vi "Untitled 1.vi"() -> ()   [LabVIEW 2023]
panel:
  in  "Restart":bool
  in  "8 8":string
  in  "7 8":string
  in  "6 8":string="2"
  in  "5 8":string="7"
  in  "8 7":string
  in  "7 7":string
  in  "6 7":string
  in  "5 7":string="8"
  in  "8 6":string
  in  "7 6":string
  in  "6 6":string
  in  "5 6":string="1"
  in  "8 5":string="5"
  in  "7 5":string
  in  "6 5":string
  in  "5 5":string
  in  "8 4":string="4"
  in  "7 4":string="3"
  in  "6 4":string="7"
  in  "5 4":string
  in  "8 3":string
  in  "7 3":string="8"
  in  "6 3":string
  in  "5 3":string="2"
  in  "8 2":string
  in  "7 2":string
  in  "6 2":string="4"
  in  "5 2":string="6"
  in  "8 1":string="1"
  in  "7 1":string="7"
  in  "6 1":string
  in  "5 1":string
  in  "8 0":string="8"
  in  "7 0":string="6"
  in  "6 0":string="9"
  in  "5 0":string
  in  "4 8":string
  in  "4 7":string="9"
  in  "4 6":string
  in  "4 5":string
  in  "4 4":string
  in  "4 3":string
  in  "4 2":string="3"
  in  "4 1":string
  in  "4 0":string
  in  "3 8":string="4"
  in  "3 7":string
  in  "3 6":string
  in  "3 5":string
  in  "3 4":string
  in  "3 3":string="6"
  in  "3 2":string="8"
  in  "3 1":string="5"
  in  "3 0":string
  in  "2 8":string
  in  "2 7":string="1"
  in  "2 6":string
  in  "2 5":string="7"
  in  "2 4":string
  in  "2 3":string
  in  "2 2":string
  in  "2 1":string
  in  "2 0":string
  in  "1 8":string="9"
  in  "1 7":string
  in  "1 6":string="3"
  in  "1 5":string
  in  "1 4":string="6"
  in  "1 3":string
  in  "1 2":string
  in  "1 1":string
  in  "1 0":string="2"
  in  "0 8":string="5"
  in  "0 7":string
  in  "0 6":string="6"
  in  "0 5":string="1"
  in  "0 4":string="9"
  in  "0 3":string="4"
  in  "0 2":string="7"
  in  "0 1":string
  in  "0 0":string
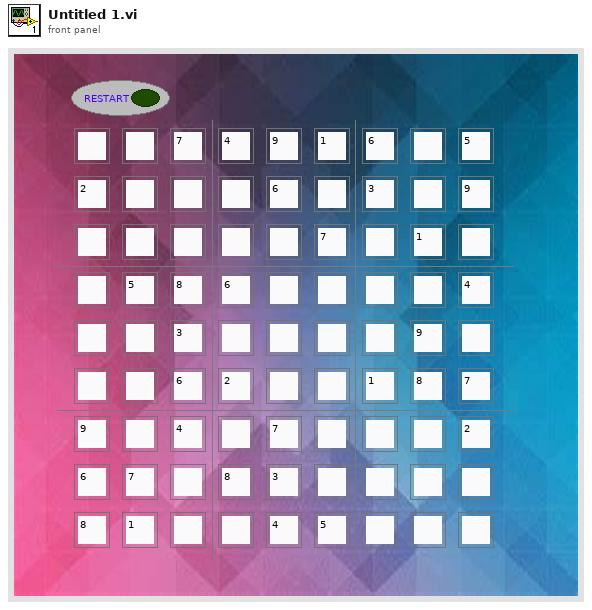
[diagram p1: front panel]
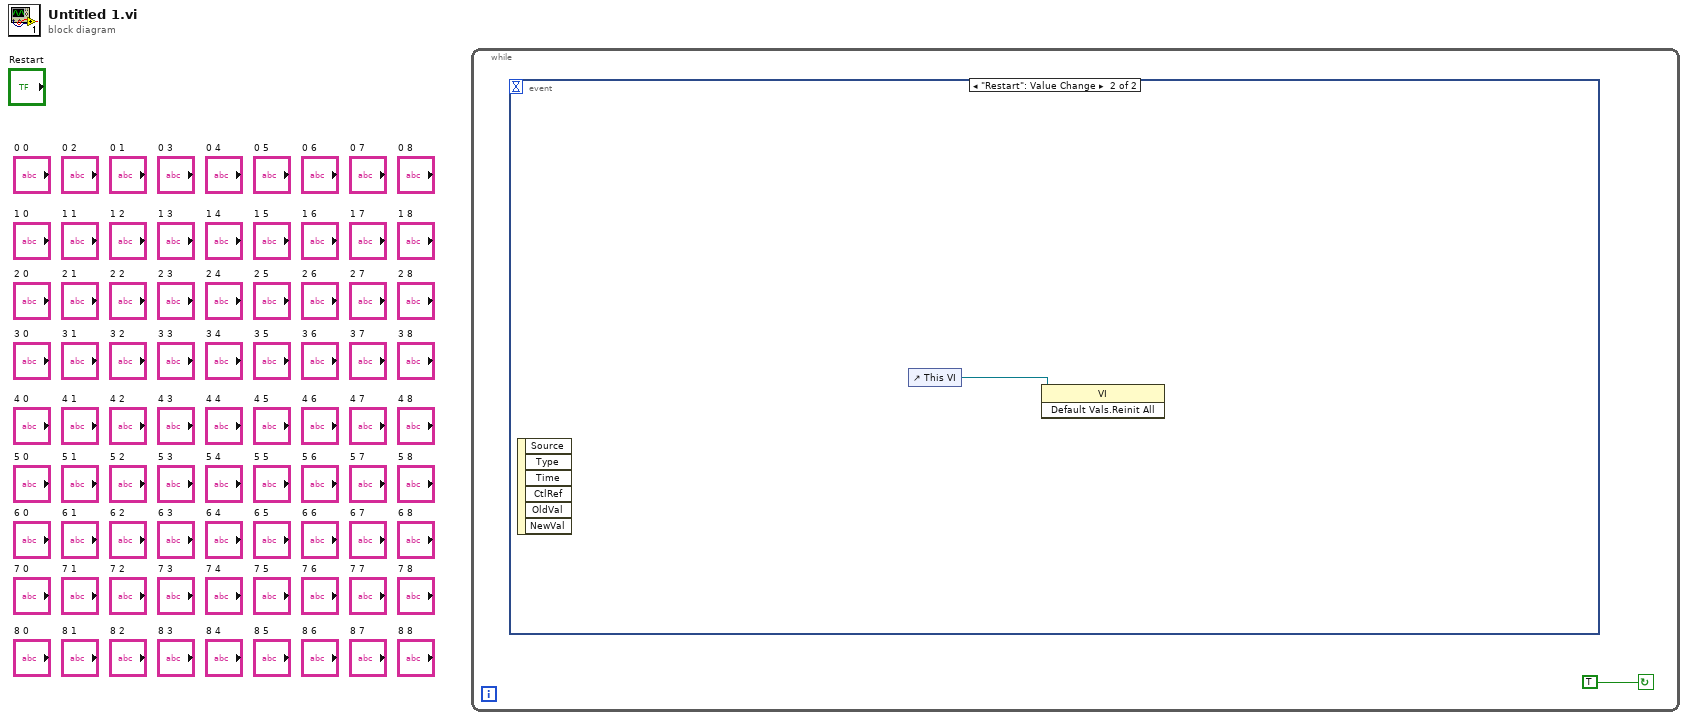
[diagram p0: block diagram]
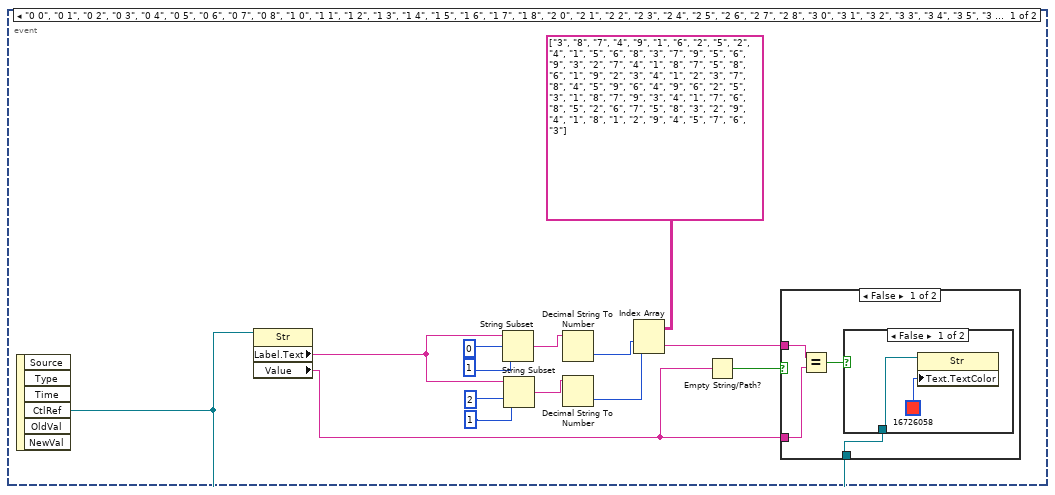
[diagram p2: hidden frame]
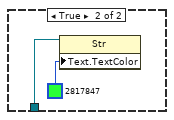
[diagram p3: hidden frame]
diagram:
  n1 = while {
    stop <- TRUE continue-if-true
    n2 = event shown="[1] \"Restart\": Value Change" {
      selector: _ -> [_ _]
      dyn-events: _ -> [_ _]
      timeout: _ -> [_ _]
      event "0 0", "0 1", "0 2", "0 3", "0 4", "0 5", "0 6", "0 7", "0 8", "1 0", "1 1", "1 2", "1 3", "1 4", "1 5", "1 6", "1 7", "1 8", "2 0", "2 1", "2 2", "2 3", "2 4", "2 5", "2 6", "2 7", "2 8", "3 0", "3 1", "3 2", "3 3", "3 4", "3 5", "3 6", "3 7", "3 8", "4 0", "4 1", "4 2", "4 3", "4 4", "4 5", "4 6", "4 7", "4 8", "5 0", "6 0", "7 0", "8 0", "5 1", "6 1", "7 1", "5 2", "6 2", "7 2", "8 2", "5 3", "6 3", "7 3", "8 3", "5 4", "6 4", "8 1", "7 4", "8 4", "5 5", "6 5", "7 5", "8 5", "5 6", "6 6", "7 6", "8 6", "5 7", "6 7", "7 7", "8 7", "5 8", "6 8", "7 8", "8 8": Value Change {
        n3 = event-data() -> ("CtlRef"=w2:refnum<vi>)  [unwired: 1 in, 5 out]
        n4 = property class="Str"(reference=w2) -> ("Label.Text"=w15:string, "Value"=w3:string)  [unwired: 1 in, 2 out]
        n5 = String Subset(string=w15, offset (0)=0, length (rest)=1) -> (substring=w9:string)
        n6 = String Subset(string=w15, offset (0)=2, length (rest)=1) -> (substring=w8:string)
        n7 = Decimal String To Number(string=w9) -> (number=w6:i32)  [unwired: 2 in, 1 out]
        n8 = Decimal String To Number(string=w8) -> (number=w7:i32)  [unwired: 2 in, 1 out]
        n9 = Index Array(array=string[][] [["3", "8", "7", "4", "9", "1", "6", "2", "5"], ["2", "4", "1", "5", "6", "8", "3", "7", "9"], ["5", "6", "9", "3", "2", "7", "4", "1", "8"], ["7", "5", "8", "6", "1", "9", "2", "3", "4"], ["1", "2", "3", "7", "8", "4", "5", "9", "6"], ["4", "9", "6", "2", "5", "3", "1", "8", "7"], ["9", "3", "4", "1", "7", "6", "8", "5", "2"], ["6", "7", "5", "8", "3", "2", "9", "4", "1"], ["8", "1", "2", "9", "4", "5", "7", "6", "3"]], index (row)=w6, index (col)=w7) -> (element=w4:string)
        n10 = Empty String/Path?(string/path=w3) -> (empty?=w5:bool)
        n11 = case shown="False" w5 {
          tunnel: w4 -> [w18 _]
          tunnel: w3 -> [w17 _]
          tunnel: w2 -> [w16 _]
          frame False {
            n12 = Equal?(x=w18, y=w17) -> (x = y?=w19:bool)
            n13 = case shown="False" w19 {
              tunnel: w16 -> [w20 w23]
              frame False {
                n14 = property class="Str"(reference=w20, "Text.TextColor"=u32 16726058) -> ()  [unwired: 1 in, 2 out]
              }
              frame True {
                n15 = property class="Str"(reference=w23, "Text.TextColor"=u32 2817847) -> ()  [unwired: 1 in, 2 out]
              }
            }
          }
          frame True {
          }
        }
      }
      event "Restart": Value Change {
        n16 = event-data() -> ()  [unwired: 1 in, 6 out]
        n17 = control-ref of="This VI"() -> (w24:refnum<vi>)
        n18 = invoke class="VI" method="Default Vals.Reinit All"(reference=w24) -> ()  [unwired: 2 in, 3 out]
      }
    }
  }
